vi "Average_Column_Values.vi"(1 "Present Values":string[][](array[string]), 2 "Present Channels":string[](array[string]), 3 "Channel operations":string[](array[string]), 4 "Channel names for operations":string[](array[string])) -> (0 "Desired Row values":string[](array[string]))   [LabVIEW 2022 SP3]
uses:
  <vilib>/Analysis/baseanly.llb/Mean (DBL).vi
  <vilib>/Analysis/NI_AALBase.lvlib
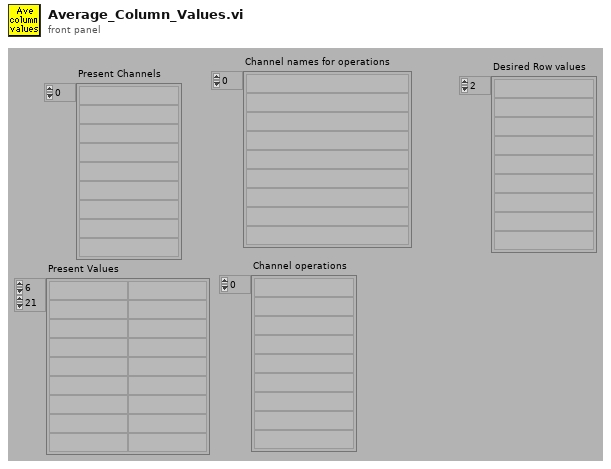
[diagram p1: front panel]
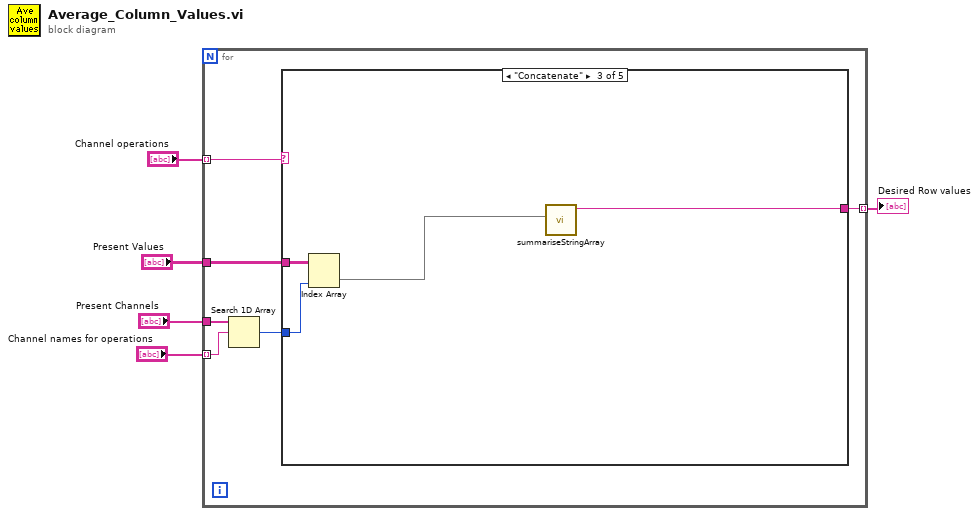
[diagram p0: block diagram]
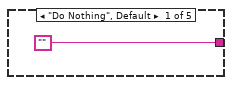
[diagram p2: hidden frame]
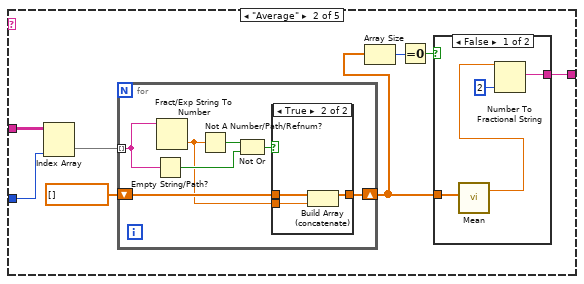
[diagram p3: hidden frame]
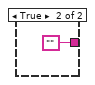
[diagram p4: hidden frame]
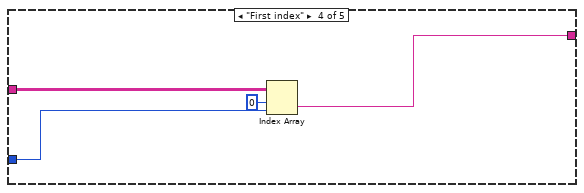
[diagram p6: hidden frame]
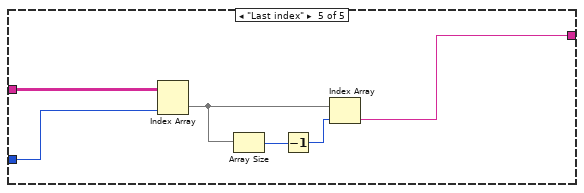
[diagram p7: hidden frame]
diagram:
  n1 = for {
    tunnel: "Channel names for operations" -> [w11] mode=indexing
    tunnel: "Present Channels" -> [w10]
    tunnel: "Channel operations" -> [w9] mode=indexing
    tunnel: "Present Values" -> [w8]
    tunnel: [w6] -> w3 mode=indexing
    n2 = Search 1D Array(1D array=w10, element=w11) -> (index of element=w7:i32)  [unwired: 1 out]
    n3 = case shown="\"Concatenate\"" w9 {
      tunnel: w8 -> [_ w20 w40 w44 w50]
      tunnel: w7 -> [_ w19 w39 w43 w49]
      tunnel: ["" w17 w38 w41 w45] -> w6
      frame "Do Nothing", Default {
      }
      frame "Average" {
        n4 = Index Array(array=w20, index (col)=w19) -> (element=w18:string[])  [unwired: 1 in]
        n5 = for {
          tunnel: w18 -> [w32] mode=indexing
          shift-right: [w28] -> w15
          shift-left: dbl[] [] -> [w27]
          n6 = Empty String/Path?(string/path=w32) -> (empty?=w30:bool)
          n7 = Fract/Exp String To Number(string=w32) -> (number=w26:dbl)  [unwired: 4 out]
          n8 = Not A Number/Path/Refnum?(number/path/refnum=w26) -> (NaN/Path/Refnum?=w31:bool)
          n9 = Not Or(1:w30, 2:w31) -> (0:w29:bool)
          n10 = case shown="True" w29 {
            tunnel: [w33 w34] -> w28
            tunnel: w27 -> [w33 w36]
            tunnel: w26 -> [_ w35]
            frame False {
            }
            frame True {
              n11 = Build Array (concatenate)(w36, w35) -> (w34:dbl[])
            }
          }
        }
        n12 = Array Size(array=w15) -> (size(s)=w14:i32)
        n13 = Equal To 0?(x=w14) -> (x = 0?=w13:bool)
        n14 = case shown="False" w13 {
          tunnel: [w23 ""] -> w17
          tunnel: w15 -> [w22 _]
          frame False {
            n15 = call-poly <vilib>:"Mean.vi"("X"=w22) -> ("mean"=w21:dbl)  [unwired: 1 out]
            n16 = Number To Fractional String(number=w21, precision (6)=i16 2) -> (F-format string=w23:string)  [unwired: 2 out]
          }
          frame True {
          }
        }
      }
      frame "Concatenate" {
        n17 = Index Array(array=w40, index (col)=w39) -> (element=w37:string[])  [unwired: 1 in]
        n18 = call "summariseStringArray.vi"("stringArray"=w37) -> ("percentagesString"=w38:string)  [unwired: 9 in, 1 out]
      }
      frame "First index" {
        n19 = Index Array(array=w44, index (row)=0, index (col)=w43) -> (element=w41:string)
      }
      frame "Last index" {
        n20 = Index Array(array=w50, index (col)=w49) -> (element=w48:string[])  [unwired: 1 in]
        n21 = Array Size(array=w48) -> (size(s)=w47:i32)
        n22 = Decrement(x=w47) -> (x-1=w46:i32)
        n23 = Index Array(array=w48, index=w46) -> (element=w45:string)
      }
    }
  }
  "Desired Row values" <- w3
